vi "Send UNSUBSCRIBE.vi"(0 "WAMP Client in":refnum<class "WAMP Client.lvclass">, 5 "error in (no error)":errorcluster, 7 "Unsubscribe Request Data":T2, 9 "Unsubscribe Requests Map (in)":T1, 11 "Subscriptions":T3) -> (4 "WAMP Client out":refnum<class "WAMP Client.lvclass">, 6 "error out":errorcluster, 10 "Unsubscribe Requests Map (out)":T1)   [LabVIEW 2020, in "wamplv.lvlib" / "WAMP Client.lvclass"]
uses:
  <userlib>/wamplv/WAMP Client/WAMP Client.lvclass
  <userlib>/wamplv/WAMP Client/TypeDef/UNSUBSCRIBE Request Data.ctl
  <userlib>/wamplv/WAMP Client/TypeDef/UNSUBSCRIBE Result.ctl
  <userlib>/wamplv/WAMP Client/TypeDef/Unsubscribe Requests Map.ctl
  <userlib>/wamplv/WAMP Client/TypeDef/Subscriptions Map.ctl
  <userlib>/wamplv/WAMP Client/TypeDef/Subscription Details.ctl
  <userlib>/wamplv/WAMP Client/TypeDef/Event Payload.ctl
  <userlib>/wamplv/WAMP Message Codes.ctl
  <userlib>/wamplv/WAMP Client/WAMP Client.lvclass/WAMP Client.ctl
  <vilib>/numeric/Random Number (Range) U64.vi
  <vilib>/numeric/sub_Random U32.vi
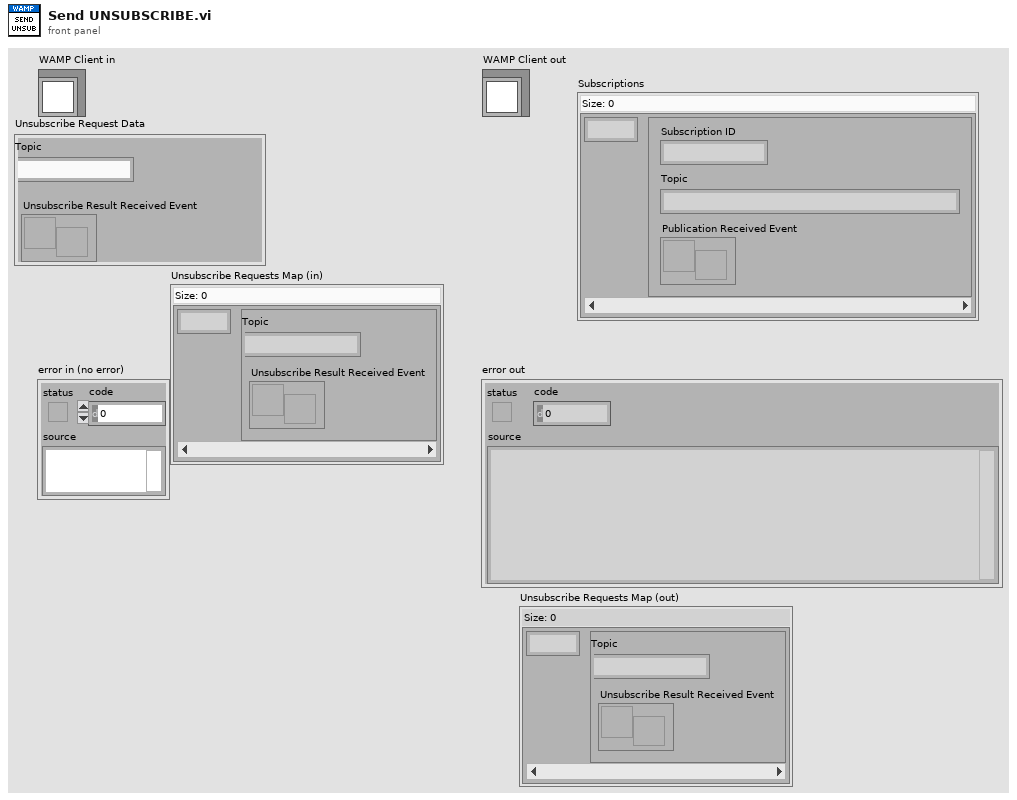
[diagram p1: front panel]
types:
  T1 = typedef "wamplv.lvlib/WAMP Client.lvclass/Unsubscribe Requests Map.ctl" = map{u32, T2}
  T2 = typedef "wamplv.lvlib/WAMP Client.lvclass/UNSUBSCRIBE Request Data.ctl" = cluster{"Topic":string, "Unsubscribe Result Received Event":refnum<user-event>}
  T3 = typedef "wamplv.lvlib/WAMP Client.lvclass/Subscriptions Map.ctl" = map{u32, T4}
  T4 = typedef "wamplv.lvlib/WAMP Client.lvclass/Subscription Details.ctl" = cluster{"Subscription ID":u32, "Topic":string, "Publication Received Event":refnum<user-event>}
  T5 = typedef "wamplv.lvlib/WAMP Client.lvclass/WAMP Message Codes.ctl" = u16
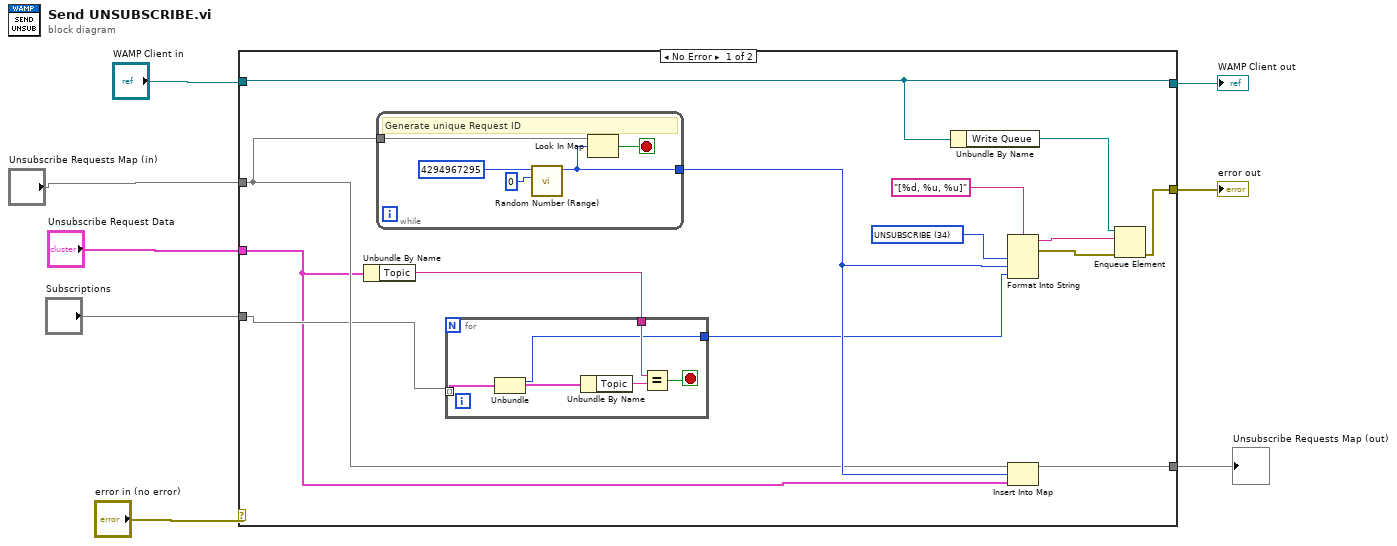
[diagram p0: block diagram]
diagram:
  n1 = case shown="No Error" "error in (no error)" {
    selector: "error in (no error)" -> [_ w36]
    tunnel: [w14 w36] -> w7
    tunnel: [w18 w35] -> w5
    tunnel: "WAMP Client in" -> [w18 w35]
    tunnel: "Unsubscribe Request Data" -> [w11 _]
    tunnel: "Unsubscribe Requests Map (in)" -> [w15 w34]
    tunnel: [w16 w34] -> w1
    tunnel: "Subscriptions" -> [w12 _]
    frame No Error {
      w19 = T5 34 items=["HELLO"=1, "WELCOME"=2, "ABORT"=3, "GOODBYE"=6, "ERROR"=8, "PUBLISH"=16, "PUBLISHED"=17, "SUBSCRIBE"=32, "SUBSCRIBED"=33, "UNSUBSCRIBE"=34, "UNSUBSCRIBED"=35, "EVENT"=36, "CALL"=48, "RESULT"=59, "REGISTER"=64, "REGISTERED"=65, "UNREGISTER"=66, "UNREGISTERED"=67, "INVOCATION"=68, "YIELD"=70] ("Message Codes")
      n2 = Unbundle By Name(w11) -> ("Topic"=w10:string)
      n3 = while {
        tunnel: w15 -> [w31]
        tunnel: [w29] -> w17
        stop <- w30 stop-if-true
        # "Generate unique Request ID"
        n4 = call-poly <vilib>:"Random Number (Range).vi"("lower bound (0)"=u32 0, "upper bound (100)"=u32 4294967295) -> ("number"=w29:u64)  [unwired: 9 in]
        n5 = Look In Map(map=w31, key=w29) -> (key not found?=w30:bool)  [unwired: 1 in, 1 out]
      }
      n6 = for {
        tunnel: w12 -> [w28] mode=indexing
        tunnel: w10 -> [w25]
        tunnel: [w23] -> w9
        stop <- w24 stop-if-true
        n7 = Unbundle(w28) -> (w23:u32, w27:T4)
        n8 = Unbundle By Name(w27) -> ("Topic"=w26:string)
        n9 = Equal?(x=w25, y=w26) -> (x = y?=w24:bool)
      }
      n10 = Unbundle By Name(w18) -> ("Write Queue"=w13:refnum<queue>)
      n11 = Format Into String(format string="[%d, %u, %u]" ("element"), w19, w17, w9) -> (resulting string=w21:string, error out=w22:errorcluster)  [unwired: 2 in]
      n12 = Insert Into Map(map in=w15, key=w17, value=w11) -> (map out=w16:T1)  [unwired: 2 out]
      n13 = Enqueue Element(queue=w13, element=w21, error in (no error)=w22) -> (error out=w14:errorcluster)  [unwired: 1 in, 2 out]
    }
    frame Error {
    }
  }
  "error out" <- w7
  "WAMP Client out" <- w5
  "Unsubscribe Requests Map (out)" <- w1
